vi "CheckElapsedTime.vi"(8 "error in (no error)":errorcluster, 11 "Enum":enum16{"Start", "Get"}(ring)=enum."Get") -> (0 "error out":errorcluster, 3 "Elapsed Time (s)":dbl)   [LabVIEW 2018]
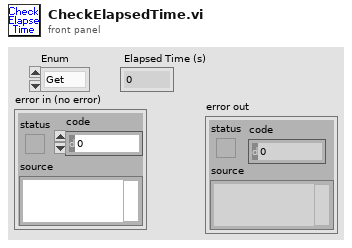
[diagram p1: front panel]
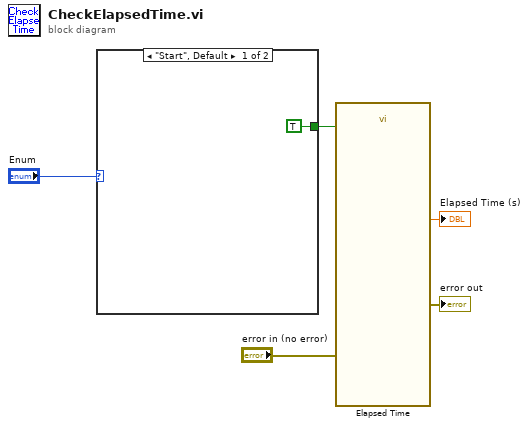
[diagram p0: block diagram]
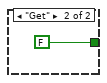
[diagram p2: hidden frame]
diagram:
  n1 = case shown="\"Start\", Default" "Enum" {
    tunnel: [TRUE ("Reset") FALSE ("Reset")] -> w4
    frame "Start", Default {
    }
    frame "Get" {
    }
  }
  n2 = call "Elapsed Time"("Reset"=w4, "error in (no error)"="error in (no error)") -> ("Elapsed Time (s)"=→"Elapsed Time (s)":dbl, "error out"=→"error out":errorcluster)  [unwired: 10 in, 6 out]
